vi "mDrive Send Command_mod1.vi"(6 "error in (no error)":errorcluster, 7 "Extra":string, 8 "Command":T1(ring), 9 "VISA resource name":refnum<visa-resource-name>="COM1") -> (0 "error out":errorcluster, 2 "read buffer":string, 3 "VISA resource name out":refnum<visa-resource-name>)   [LabVIEW 2009]
uses:
  Instance           1 28Saved   Applied Send Command .vi
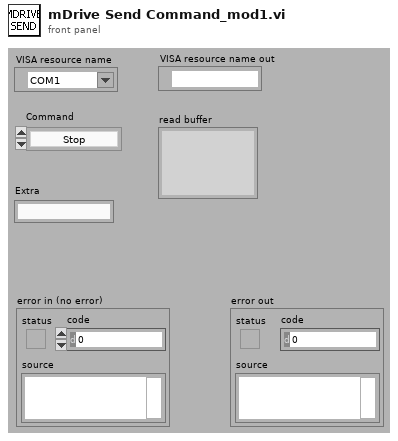
[diagram p1: front panel]
types:
  T1 = enum16{"Stop", "Reset", "Run Current", "Holding Current", "Accel Rate", "Decel Rate", "Move to Relative Position", "Move to Absolute Position", "Prtint Position", "Print Encorder", "Print Velocity Maximum", "Print Velocity", "Microstep Resolution", "Max Velocity"}
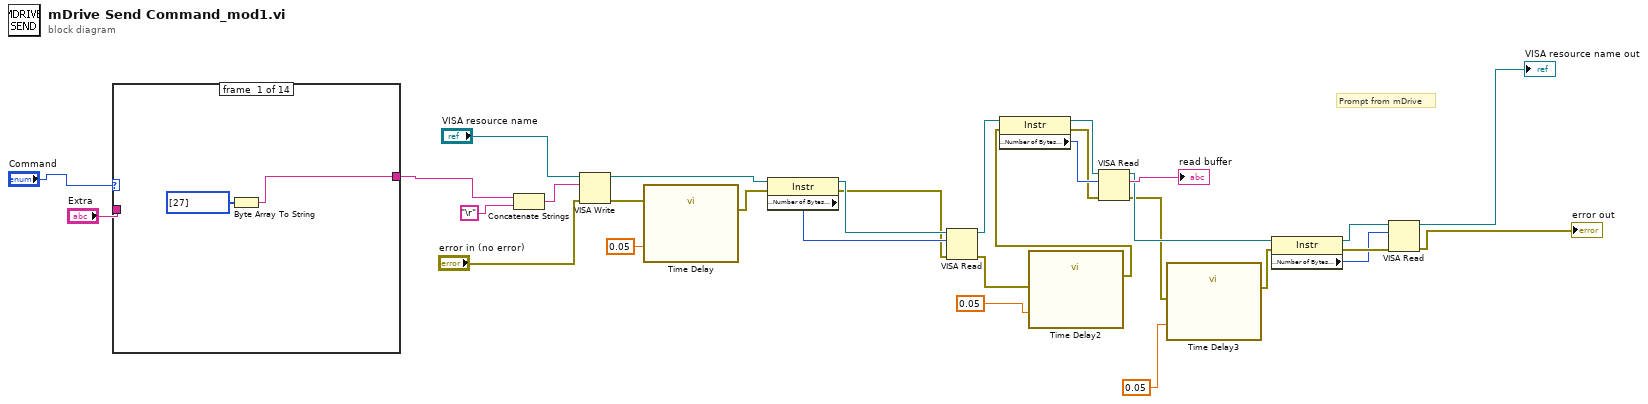
[diagram p0: block diagram]
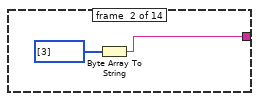
[diagram p2: hidden frame]
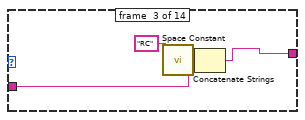
[diagram p3: hidden frame]
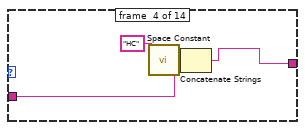
[diagram p4: hidden frame]
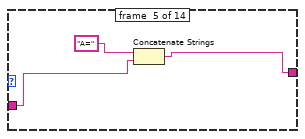
[diagram p5: hidden frame]
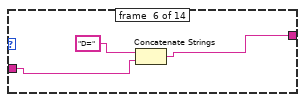
[diagram p6: hidden frame]
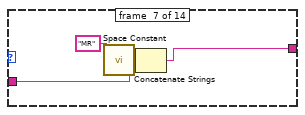
[diagram p7: hidden frame]
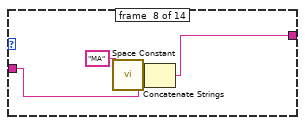
[diagram p8: hidden frame]
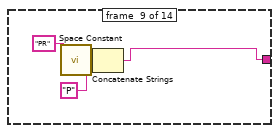
[diagram p9: hidden frame]
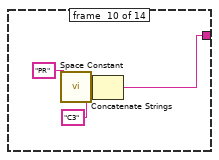
[diagram p10: hidden frame]
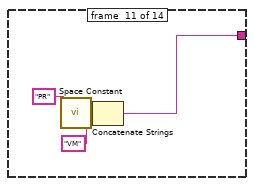
[diagram p11: hidden frame]
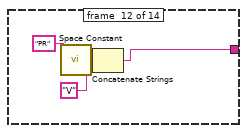
[diagram p12: hidden frame]
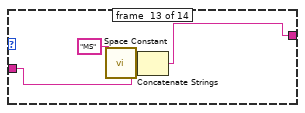
[diagram p13: hidden frame]
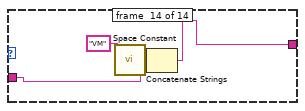
[diagram p14: hidden frame]
diagram:
  # "Prompt from mDrive"
  n1 = case shown="\"Print Velocity\"" "Command" {
    tunnel: "Extra" -> [_ _ w37 w41 w44 w48 w51 w55 _ _ _ _ w75 w79]
    tunnel: [w32 w35 w38 w42 w45 w47 w50 w54 w59 w62 w66 w70 w74 w78] -> w20
    frame #0 {
      n2 = Byte Array To String(unsigned byte array=u8[] [27]) -> (string=w32:string)
    }
    frame #1 {
      n3 = Byte Array To String(unsigned byte array=u8[] [3]) -> (string=w35:string)
    }
    frame #2 {
      n4 = call <vilib>:"Space Constant.vi"() -> ("String"=w36:string)
      n5 = Concatenate Strings("RC", w36, w37) -> (w38:string)
    }
    frame #3 {
      n6 = call <vilib>:"Space Constant.vi"() -> ("String"=w40:string)
      n7 = Concatenate Strings("HC", w40, w41) -> (w42:string)
    }
    frame #4 {
      n8 = Concatenate Strings("A=", w44) -> (w45:string)
    }
    frame #5 {
      n9 = Concatenate Strings("D=", w48) -> (w47:string)
    }
    frame #6 {
      n10 = call <vilib>:"Space Constant.vi"() -> ("String"=w52:string)
      n11 = Concatenate Strings("MR", w52, w51) -> (w50:string)
    }
    frame #7 {
      n12 = call <vilib>:"Space Constant.vi"() -> ("String"=w56:string)
      n13 = Concatenate Strings("MA", w56, w55) -> (w54:string)
    }
    frame #8 {
      n14 = call <vilib>:"Space Constant.vi"() -> ("String"=w60:string)
      n15 = Concatenate Strings("PR", w60, "P") -> (w59:string)
    }
    frame #9 {
      n16 = call <vilib>:"Space Constant.vi"() -> ("String"=w64:string)
      n17 = Concatenate Strings("PR", w64, "C3") -> (w62:string)
    }
    frame #10 {
      n18 = call <vilib>:"Space Constant.vi"() -> ("String"=w68:string)
      n19 = Concatenate Strings("PR", w68, "VM") -> (w66:string)
    }
    frame #11 {
      n20 = call <vilib>:"Space Constant.vi"() -> ("String"=w72:string)
      n21 = Concatenate Strings("PR", w72, "V") -> (w70:string)
    }
    frame #12 {
      n22 = call <vilib>:"Space Constant.vi"() -> ("String"=w76:string)
      n23 = Concatenate Strings("MS", w76, w75) -> (w74:string)
    }
    frame #13 {
      n24 = call <vilib>:"Space Constant.vi"() -> ("String"=w80:string)
      n25 = Concatenate Strings("VM", w80, w79) -> (w78:string)
    }
  }
  n26 = Concatenate Strings(w20, "\r") -> (w28:string)
  n27 = VISA Write(VISA resource name="VISA resource name", write buffer=w28, error in (no error)="error in (no error)") -> (VISA resource name out=w31:refnum<visa-resource-name>, error out=w26:errorcluster)  [unwired: 1 out]
  n28 = call "Time Delay"("error in (no error)"=w26, "Delay Time (s)"=0.05) -> ("error out"=w25:errorcluster)  [unwired: 9 in]
  n29 = property class="Instr"(reference=w31, error in=w25) -> (reference out=w19:refnum<visa-resource-name>, error out=w17:errorcluster, "Serial Settings:Number of Bytes at Serial Port"=w18:u32)
  n30 = VISA Read(VISA resource name=w19, byte count=w18, error in (no error)=w17) -> (VISA resource name out=w16:refnum<visa-resource-name>, error out=w6:errorcluster)  [unwired: 2 out]
  n31 = call "Time Delay2"("error in (no error)"=w6, "Delay Time (s)"=0.05) -> ("error out"=w5:errorcluster)  [unwired: 9 in]
  n32 = property class="Instr"(reference=w16, error in=w5) -> (reference out=w14:refnum<visa-resource-name>, error out=w13:errorcluster, "Serial Settings:Number of Bytes at Serial Port"=w15:u32)
  n33 = VISA Read(VISA resource name=w14, byte count=w15, error in (no error)=w13) -> (VISA resource name out=w12:refnum<visa-resource-name>, read buffer=→"read buffer":string, error out=w3:errorcluster)  [unwired: 1 out]
  n34 = call "Time Delay3"("error in (no error)"=w3, "Delay Time (s)"=0.05) -> ("error out"=w2:errorcluster)  [unwired: 9 in]
  n35 = property class="Instr"(reference=w12, error in=w2) -> (reference out=w11:refnum<visa-resource-name>, error out=w10:errorcluster, "Serial Settings:Number of Bytes at Serial Port"=w7:u32)
  n36 = VISA Read(VISA resource name=w11, byte count=w7, error in (no error)=w10) -> (VISA resource name out=→"VISA resource name out":refnum<visa-resource-name>, error out=→"error out":errorcluster)  [unwired: 2 out]
